vi "SineFit.vi"(3 "initial parameters":dbl[](array[numeric]), 4 "model description":T1, 5 "data template":cluster{dbl[], dbl[]}) -> (0 "residuals":cluster{dbl[], dbl[]}, 1 "best fit parameters":dbl[](array[numeric]), 2 "chart and fit":cluster{dbl[], "best nonlinear fit":dbl[]}[](array[cluster]))   [LabVIEW 2011]
doc: "Performs a least squares best fot for taking out the one-per-revolution out-of-center effect."
uses:
  <vilib>/gmath/NumericalOptimization/Nonlinear Curve Fit LM formula string.vi
  <vilib>/gmath/NI_Gmath.lvlib
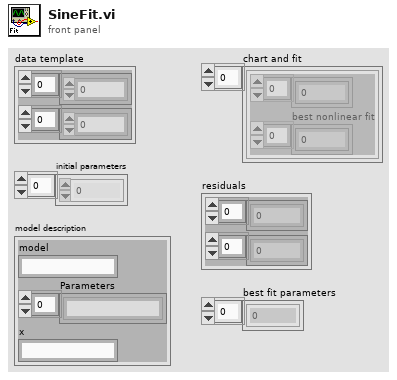
[diagram p1: front panel]
types:
  T1 = cluster{"model":string, "Parameters":string[], "x":string}
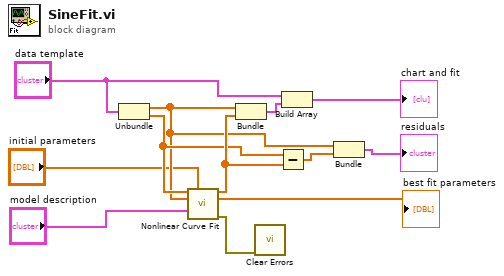
[diagram p0: block diagram]
diagram:
  n1 = Unbundle("data template") -> (w7:dbl[], w9:dbl[])
  n2 = call-poly <vilib>:"Nonlinear Curve Fit.vi"("Y"=w9, "initial parameters"="initial parameters", "X"=w7, "model description"="model description") -> ("best nonlinear fit"=w10:dbl[], "best fit parameters"=→"best fit parameters":dbl[], "error out"=w12:errorcluster)  [unwired: 7 in, 2 out]
  n3 = Bundle(w7, "best nonlinear fit"=w10) -> (w5:cluster{dbl[], "best nonlinear fit":dbl[]})  [unwired: 1 in]
  n4 = call <vilib>:"Clear Errors.vi"("error in (no error)"=w12) -> ()  [unwired: 6 in, 1 out]
  n5 = Subtract(x=w9, y=w10) -> (x-y=w8:dbl[])
  n6 = Build Array("data template", w5) -> (→"chart and fit":cluster{dbl[], "best nonlinear fit":dbl[]}[])
  n7 = Bundle(w7, w8) -> (→"residuals":cluster{dbl[], dbl[]})  [unwired: 1 in]
